vi "HTML Front Panel Save.vi"(5 "url":string, 7 "title":string="bd.html", 8 "error in":errorcluster, 10 "path":path, 11 "vi ref":refnum<vi>) -> (0 "error out":errorcluster, 2 "path out":path, 3 "vi ref out":refnum<vi>)   [LabVIEW 2014, in "lvprj2html.lvlib"]
uses:
  lvprj2html.lvlib
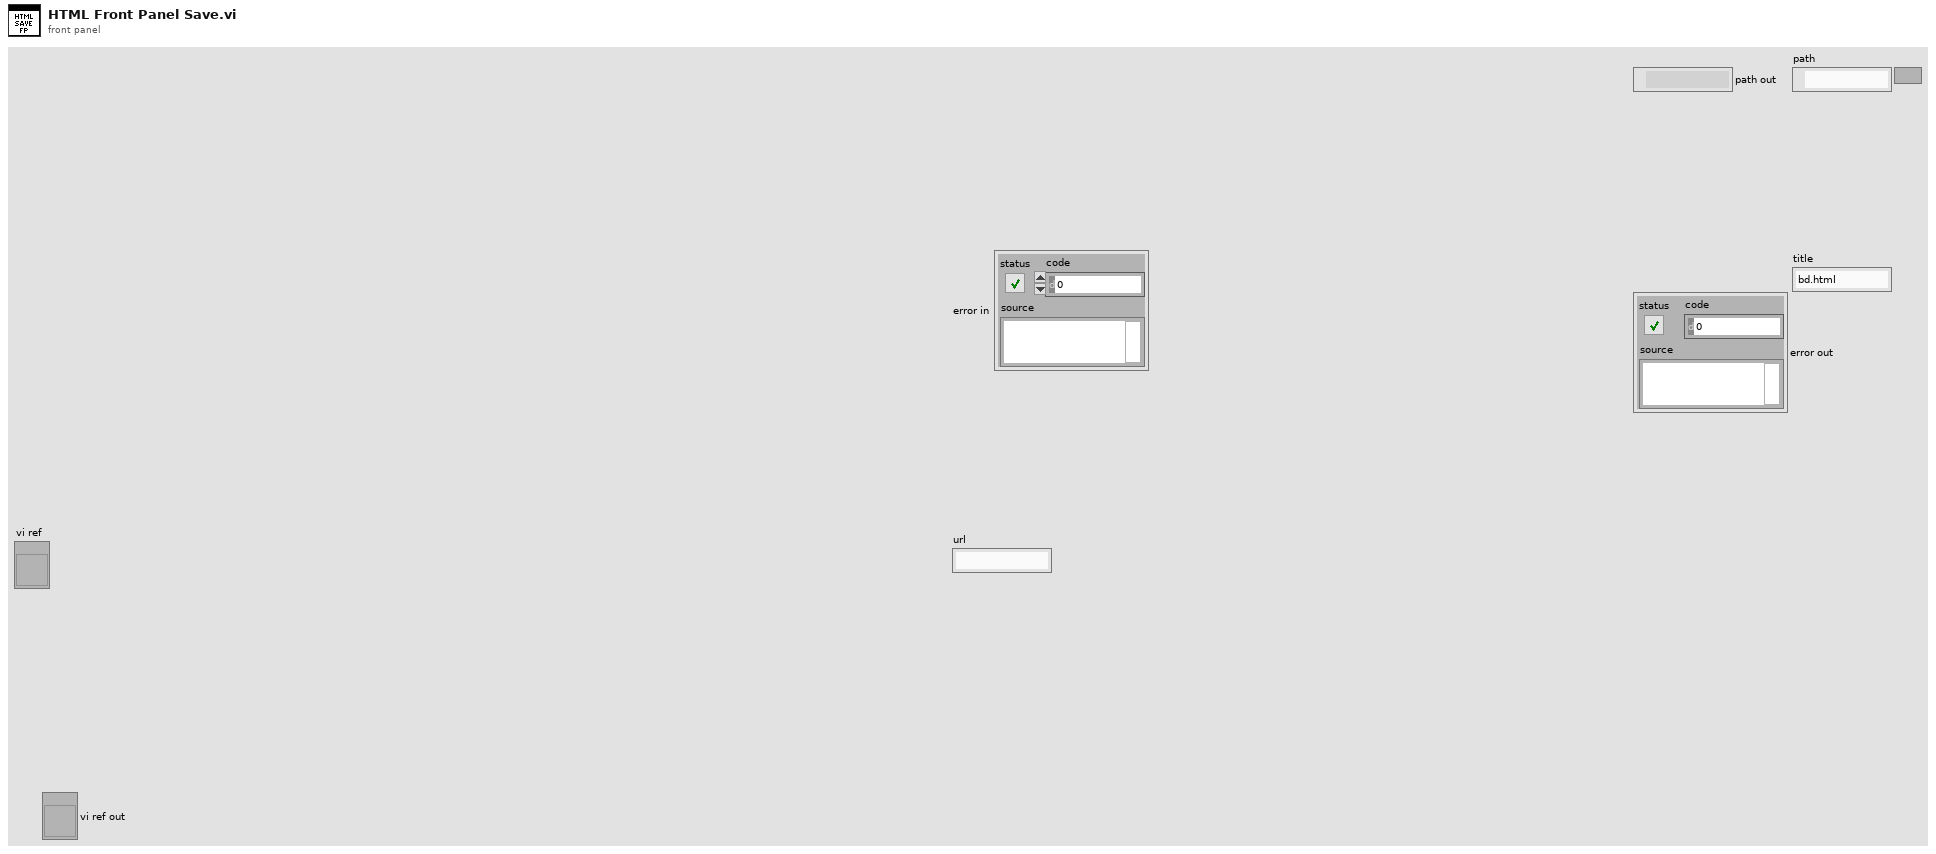
[diagram p1: front panel]
types:
  T1 = enum16{"open", "replace", "create", "open or create", "replace or create", "replace or create with confirmation"}
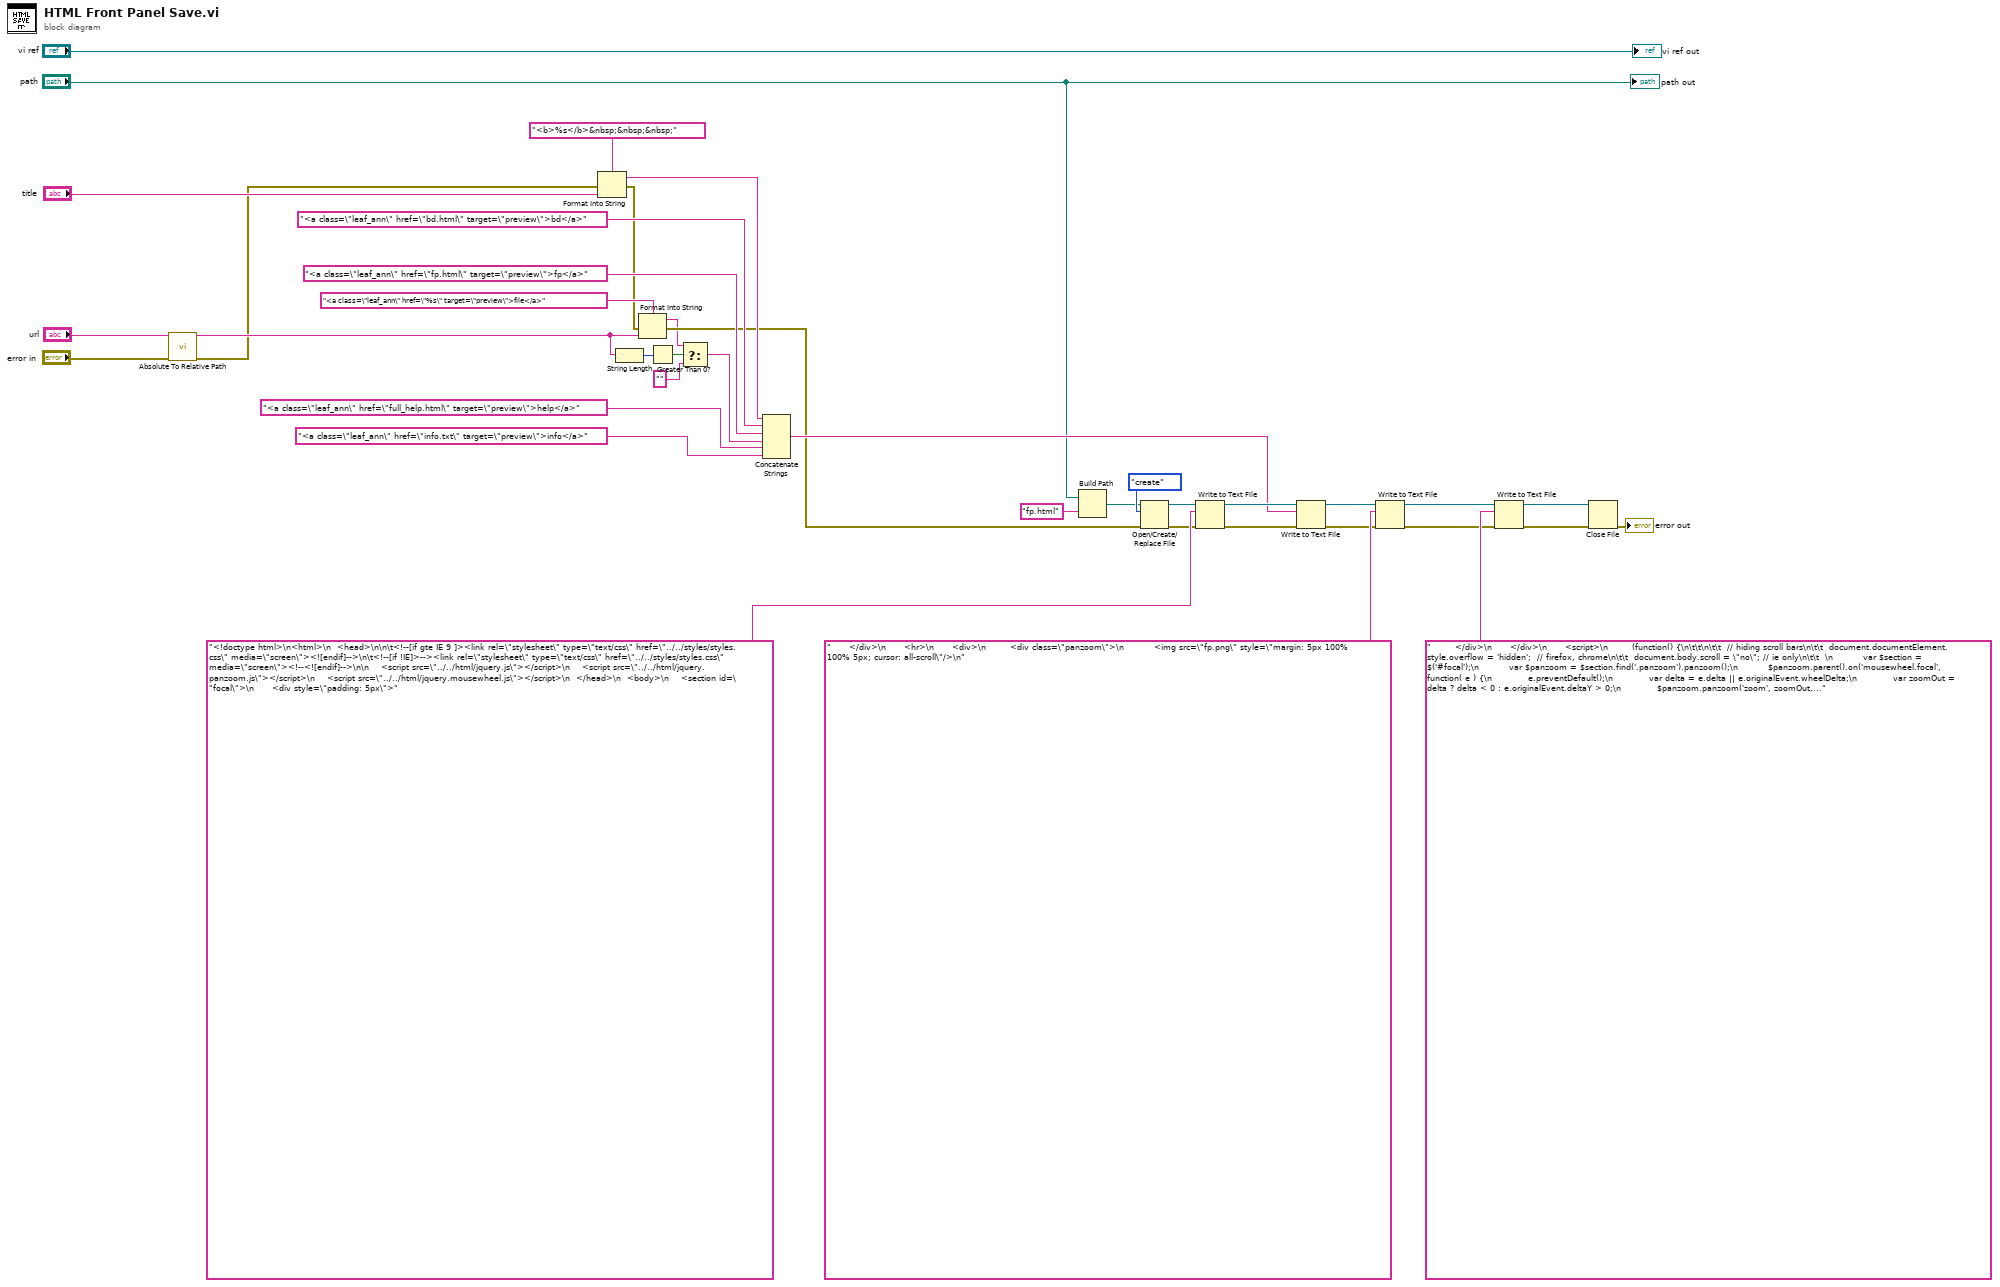
[diagram p0: block diagram]
diagram:
  n1 = call "Absolute To Relative Path.vi"("url in"="url", "error in (no error)"="error in") -> ("url out"=w3:string, "error out"=w1:errorcluster)  [unwired: 12 in]
  n2 = Format Into String(format string="<b>%s</b>&nbsp;&nbsp;&nbsp;", error in=w1, "title") -> (resulting string=w37:string, error out=w12:errorcluster)  [unwired: 1 in]
  n3 = String Length(string=w3) -> (length=w9:i32)
  n4 = Format Into String(format string="<a class=\"leaf_ann\" href=\"%s\" target=\"preview\">file</a>" ("text"), error in=w12, w3) -> (resulting string=w7:string, error out=w11:errorcluster)  [unwired: 1 in]
  n5 = Greater Than 0?(x=w9) -> (x > 0?=w8:bool)
  n6 = Select(t=w7, s=w8, f="") -> (s? t:f=w6:string)
  n7 = Concatenate Strings(w37, "<a class=\"leaf_ann\" href=\"bd.html\" target=\"preview\">bd</a>" ("text"), "<a class=\"leaf_ann\" href=\"fp.html\" target=\"preview\">fp</a>" ("text"), w6, "<a class=\"leaf_ann\" href=\"full_help.html\" target=\"preview\">help</a>" ("text"), "<a class=\"leaf_ann\" href=\"info.txt\" target=\"preview\">info</a>" ("text")) -> (w20:string)
  n8 = Build Path(base path="path", name or relative path="fp.html") -> (appended path=w29:path)
  n9 = Open/Create/Replace File(file path (use dialog)=w29, error in=w11, operation (0:open)=T1."create") -> (refnum out=w31:refnum<file>, error out=w13:errorcluster)  [unwired: 3 in, 1 out]
  n10 = Write to Text File(file (use dialog)=w31, text="<!doctype html>\n<html>\n  <head>\n\n\t<!--[if gte IE 9 ]><link rel=\"stylesheet\" type=\"text/css\" href=\"../../styles/styles.css\" media=\"screen\"><![endif]-->\n\t<!--[if !IE]>--><link rel=\"stylesheet\" type=\"text/css\" href=\"../../styles/styles.css\" media=\"screen\"><!--<![endif]-->\n\n    <script src=\"../../html/jquery.js\"></script>\n    <script src=\"../../html/jquery.panzoom.js\"></script>\n    <script src=\"../../html/jquery.mousewheel.js\"></script>\n  </head>\n  <body>\n    <section id=\"focal\">\n      <div style=\"padding: 5px\">", error in=w13) -> (refnum out=w25:refnum<file>, error out=w14:errorcluster)  [unwired: 1 in, 1 out]
  n11 = Write to Text File(file (use dialog)=w25, text=w20, error in=w14) -> (refnum out=w24:refnum<file>, error out=w15:errorcluster)  [unwired: 1 in, 1 out]
  n12 = Write to Text File(file (use dialog)=w24, text="      </div>\n      <hr>\n      <div>\n        <div class=\"panzoom\">\n          <img src=\"fp.png\" style=\"margin: 5px 100% 100% 5px; cursor: all-scroll\"/>\n", error in=w15) -> (refnum out=w21:refnum<file>, error out=w16:errorcluster)  [unwired: 1 in, 1 out]
  n13 = Write to Text File(file (use dialog)=w21, text="        </div>\n      </div>\n      <script>\n        (function() {\n\t\t\n\t\t  // hiding scroll bars\n\t\t  document.documentElement.style.overflow = 'hidden';  // firefox, chrome\n\t\t  document.body.scroll = \"no\"; // ie only\n\t\t  \n          var $section = $('#focal');\n          var $panzoom = $section.find('.panzoom').panzoom();\n          $panzoom.parent().on('mousewheel.focal', function( e ) {\n            e.preventDefault();\n            var delta = e.delta || e.originalEvent.wheelDelta;\n            var zoomOut = delta ? delta < 0 : e.originalEvent.deltaY > 0;\n            $panzoom.panzoom('zoom', zoomOut, {\n              increment: 0.1,\n\t\t\t  minScale: 0.2,\n\t\t\t  maxScale: 1,\n              animate: true,\n              focal: e\n            });\n          });\n        })();\n      </script>\n    </section>\n\n\n  </body>\n</html>", error in=w16) -> (refnum out=w27:refnum<file>, error out=w17:errorcluster)  [unwired: 1 in, 1 out]
  n14 = Close File(refnum=w27, error in=w17) -> (error out=→"error out":errorcluster)  [unwired: 1 out]
  "path out" <- "path"
  "vi ref out" <- "vi ref"
